vi "RFID card detection and reading RFID.vi"(8 "error in":errorcluster) -> (0 "error out":errorcluster, 2 "Pass/Fail":bool, 3 "RFID string":string caption="read string")   [LabVIEW 2009]
uses:
  Digit IO PCI 6503/Digit IO control.ctl
  Global/Global 1.vi
  <vilib>/Instr/_visa.llb/VISA Configure Serial Port (Instr).vi
panel:
  out "read string":string
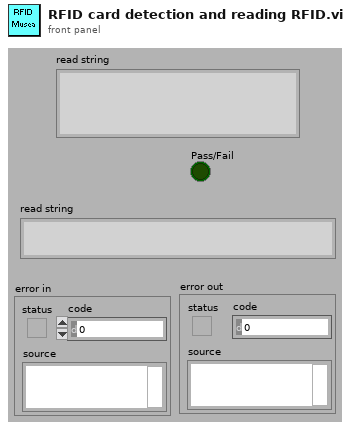
[diagram p1: front panel]
types:
  T1 = typedef "Digit IO control.ctl" = enum16{"Pull X1_4 Low", "Disconnect Pull X1_4 Low", "Down Cylinder", "Disconnect Down Cylinder", "Load X1_1_5", "Disconnect Load X1_1_5", "Measu X1_1_5", "Disconnect Measu X1_1_5", "Measu Z1_1_5", "Disconnect Measu Z1_1_5", "Power X1_1", "Disconnect Power X1_1", "RS232 Power", "Disconnect RS232 Power", "Card Cylinder", "Disconnect Card Cylinder", "Fail LED", "Disconnect Fail LED", "LCA Power", "Disconnect LCA Power", "BeyondCylinderDowndigit", "Disconnect BeyondCylinderDowendigit", "Frequency", "Disconnect Frequency", "Measu Current", "Disconnect Measu Current", "Measu current_1", "Disconnect Measu current_1", "Digit ALL", "Disconnect Digit ALL", "PASS LED", "Disconnect PASS LED", "Load Z1_1_3", "Disconnect Load Z1_1_3", "RS232 Connect", "Disconnect RS232 Connect", "Power Z1_7", "Disconnect Power Z1_7", "Pull Z_1_5  low", "Disconnect Pull Z_1_5  low", "Connect LCA_1", "Disconnect LCA_1", "short LCA", "Disconnect short LCA", "PT100", "Disconnect PT100", "NO connect", "Disconnect NO connect"}
  T2 = cluster{"VHEATFUSENOLOADMIN":string, "VHEATFUSELOADMAX":string, "VOVERRIDEDIODEMIN":string, "TDIFFMAX":string, "MEASFREQMAX":string, "MEASFREQMIN":string, "VOVER":string, "VMIDDLE":string, "VUNDER":string, "VNORESET":string, "VRESET":string, "WAITPING":string, "LRFID":string, "RFIDUID":string, "EXTEESIZE":string, "LCUTYPE":string, "LCUSUBTYPE":string, "TEVN":string, "BOOTVER":string, "APPVER":string, "ISLEEPMAX":string, "TSLEEP":string, "APPWAIT":string, "DBWAIT":string}
  T3 = cluster{"People":string, "product  number":string, "Test time":string, "VHeatFuse_noload":string, "VHeatFuse_load":string, "VoverrideDiode":string, "Test firmware upload via X1":string, "TemperAddress":string, "Troom":string, "TLCU":string, "Adjustment factor":string, "MeasuredFreq":string, "I2C communication":string, "Light-emitting diode on Z2":string, "Battery warning/inhibit":string, "Reset by IC10":string, "External EEPROM":string, "RFID card detection and reading RFID":string, "Production parameters in internal EEPROM":string, "Current consumption in sleep mode":string, "Application and database upload":string, "Test result":string, "Table head[22]":string, "Table head[23]":string}
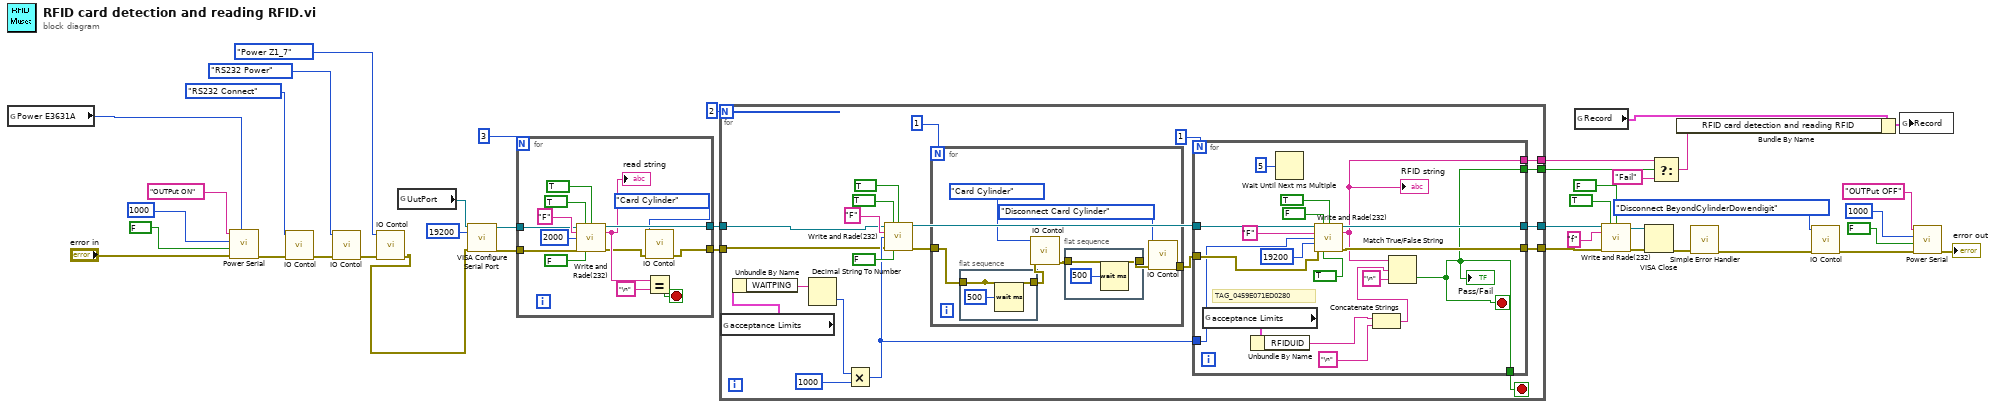
[diagram p0: block diagram]
diagram:
  n1 = global read "Global 1.vi" "Power E3631A"() -> (w17:i32)
  n2 = call "Power Serial.vi"("VISA Resource Address"=w17, "error in (no error)"="error in", "Rd?"=FALSE, "Delay"=1000, "IN"="OUTPut ON" ("In")) -> ("error out"=w14:errorcluster)  [unwired: 6 out]
  n3 = call "IO Contol.vi"("error in"=w14, "IO Operation"=Digit_IO_control."RS232 Connect" ("Enum")) -> ("error out"=w15:errorcluster)  [unwired: 9 out]
  n4 = call "IO Contol.vi"("error in"=w15, "IO Operation"=Digit_IO_control."RS232 Power" ("Enum")) -> ("error out"=w16:errorcluster)  [unwired: 9 out]
  n5 = call "IO Contol.vi"("error in"=w16, "IO Operation"=Digit_IO_control."Power Z1_7" ("Enum")) -> ("error out"=w4:errorcluster)  [unwired: 9 out]
  n6 = global read "Global 1.vi" "UutPort"() -> (w19:refnum<visa-resource-name>)
  n7 = call-poly "VISA Configure Serial Port"("VISA resource name"=w19, "baud rate (9600)"=u32 19200, "error in (no error)"=w4) -> ("VISA resource name out"=w10:refnum<visa-resource-name>, "error out"=w9:errorcluster)  [unwired: 3 in, 8 out]
  n8 = for {
    N: 3 -> [_]
    tunnel: w10 -> [w50]
    tunnel: w9 -> [w49]
    tunnel: [w43] -> w8
    tunnel: [w48] -> w7
    stop <- w46 stop-if-true
    n9 = call "Write and Rade(232).vi"("VISA resource name in"=w50, "write"=TRUE, "read"=TRUE, "string to write"="F", "ms delay"=u32 2000 ("millisecond multiple"), "error in"=w49, "change baud rate(read)"=FALSE) -> ("VISA resource name out"=w48:refnum<visa-resource-name>, "read string"=w45:string, "error out"=w44:errorcluster)  [unwired: 1 in, 5 out]
    "read string" <- w45
    n10 = call "IO Contol.vi"("error in"=w44, "IO Operation"=Digit_IO_control."Card Cylinder" ("Enum")) -> ("error out"=w43:errorcluster)  [unwired: 9 out]
    n11 = Equal?(x=w45, y="\n") -> (x = y?=w46:bool)
  }
  n12 = for {
    N: 2 -> [_]
    tunnel: w8 -> [w56]
    tunnel: w7 -> [w57]
    tunnel: [w75] -> w33
    tunnel: [w69] -> w32
    tunnel: [w74] -> w24
    tunnel: [w73] -> w22
    stop <- w71 stop-if-true
    n13 = global read "Global 1.vi" "acceptance Limits"() -> (w62:T2)
    n14 = Unbundle By Name(w62) -> ("WAITPING"=w61:string)
    n15 = Decimal String To Number(string=w61) -> (number=w60:i32)  [unwired: 3 out]
    n16 = Multiply(x=w60, y=1000) -> (x*y=w58:i32)
    n17 = call "Write and Rade(232).vi"("VISA resource name in"=w57, "write"=TRUE, "read"=TRUE, "string to write"="F", "ms delay"=w58, "error in"=w56, "change baud rate(read)"=FALSE) -> ("VISA resource name out"=w76:refnum<visa-resource-name>, "error out"=w68:errorcluster)  [unwired: 1 in, 6 out]
    n18 = for {
      N: 1 -> [_]
      tunnel: [w81] -> w70
      tunnel: w68 -> [w78]
      n19 = flat-sequence {
        tunnel: [w84] -> w77
        tunnel: [w84] -> _
        tunnel: w78 -> [w84]
        frame #0 {
          n20 = Wait (ms)(milliseconds to wait=u32 500) -> ()  [unwired: 1 out]
        }
      }
      n21 = call "IO Contol.vi"("error in"=w77, "IO Operation"=Digit_IO_control."Card Cylinder" ("Enum")) -> ("error out"=w82:errorcluster)  [unwired: 9 out]
      n22 = flat-sequence {
        tunnel: [w86] -> w80
        tunnel: w82 -> [w86]
        frame #0 {
          n23 = Wait (ms)(milliseconds to wait=u32 500) -> ()  [unwired: 1 out]
        }
      }
      n24 = call "IO Contol.vi"("error in"=w80, "IO Operation"=Digit_IO_control."Disconnect Card Cylinder" ("Enum")) -> ("error out"=w81:errorcluster)  [unwired: 9 out]
    }
    n25 = for {
      N: 1 -> [_]
      tunnel: [w99] -> w71
      tunnel: w76 -> [w104]
      tunnel: [w103] -> w75
      tunnel: [w102] -> w69
      tunnel: w70 -> [w101]
      tunnel: [w100] -> w74
      tunnel: [w99] -> w73
      tunnel: w58 -> [w93]
      stop <- w99 stop-if-true
      # "TAG_0459E071ED0280"
      n26 = global read "Global 1.vi" "acceptance Limits"() -> (w89:T2)
      n27 = Unbundle By Name(w89) -> ("RFIDUID"=w88:string)
      n28 = Wait Until Next ms Multiple(millisecond multiple=u32 5) -> ()  [unwired: 1 out]
      n29 = call "Write and Rade(232).vi"("VISA resource name in"=w104, "write"=FALSE, "read"=TRUE ("write"), "string to write"="F", "ms delay"=w93, "baud rate(read)"=u32 19200, "error in"=w101, "change baud rate(read)"=TRUE) -> ("VISA resource name out"=w103:refnum<visa-resource-name>, "read string"=w100:string, "error out"=w102:errorcluster)  [unwired: 5 out]
      "RFID string" <- w100
      n30 = Concatenate Strings(w88, "\n" ("false string")) -> (w90:string)
      n31 = Match True/False String(2:"\n" ("false string"), 3:w90, 4:w100) -> (0:w99:bool)  [unwired: 1 out]
      "Pass/Fail" <- w99
    }
  }
  n32 = global read "Global 1.vi" "Record"() -> (w26:T3)
  n33 = call "Write and Rade(232).vi"("VISA resource name in"=w33, "write"=TRUE, "read"=FALSE, "string to write"="f", "error in"=w32) -> ("VISA resource name out"=w27:refnum<visa-resource-name>, "error out"=w29:errorcluster)  [unwired: 3 in, 6 out]
  n34 = VISA Close(VISA resource name=w27, error in (no error)=w29) -> (error out=w28:errorcluster)
  n35 = Select(t=w24, s=w22, f="Fail") -> (s? t:f=w21:string)
  n36 = Bundle By Name(cluster=w26, "RFID card detection and reading RFID"=w21) -> (w25:T3)
  n37 = call <vilib>:"Simple Error Handler.vi"("error in (no error)"=w28) -> ("error out"=w35:errorcluster)  [unwired: 1 in, 7 out]
  n38 = call "IO Contol.vi"("error in"=w35, "IO Operation"=Digit_IO_control."Disconnect BeyondCylinderDowendigit" ("Enum")) -> ("error out"=w38:errorcluster)  [unwired: 9 out]
  n39 = global write "Global 1.vi" "Record"(w25) -> ()
  n40 = call "Power Serial.vi"("error in (no error)"=w38, "Rd?"=FALSE, "Delay"=1000, "IN"="OUTPut OFF" ("In")) -> ("error out"=→"error out":errorcluster)  [unwired: 1 in, 6 out]
